vi "DataLog FGV.vi"(7 "Method":T1=enum."Add One Record", 8 "error in (no error)":errorcluster, 10 "length":u16, 11 "New Record":string[](array[string])) -> (0 "error out":errorcluster, 2 "log to file":string[][](array[string]), 3 "Speed Log":string[][](table))   [LabVIEW 2018]
uses:
  Ctls/DatabaseCmd.ctl
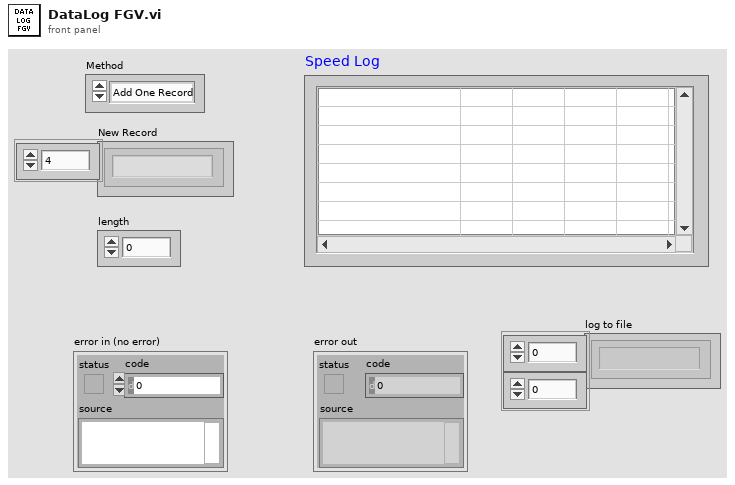
[diagram p1: front panel]
types:
  T1 = typedef "DatabaseCmd.ctl" = enum16{"Insert Table Title", "Add One Record", "Delete Record", "Get Table Records", "Clear"}
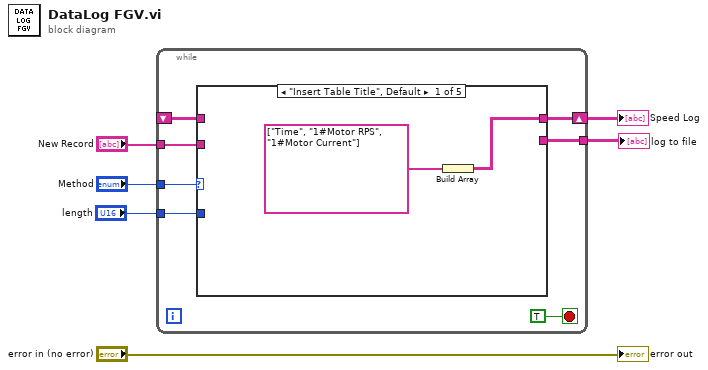
[diagram p0: block diagram]
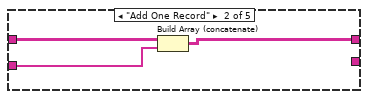
[diagram p2: hidden frame]
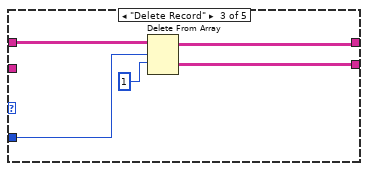
[diagram p3: hidden frame]
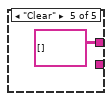
[diagram p5: hidden frame]
diagram:
  n1 = while {
    tunnel: "Method" -> [w12]
    shift-right: [w10] -> w6
    shift-left: _ -> [w11]
    tunnel: "New Record" -> [w9]
    tunnel: "length" -> [w8]
    tunnel: [w7] -> w1
    stop <- TRUE stop-if-true
    n2 = case shown="\"Insert Table Title\", Default" w12 {
      tunnel: w11 -> [_ w16 w23 w24 _]
      tunnel: [w14 w17 w22 w24 string[][] []] -> w10
      tunnel: w9 -> [_ w18 _ _ _]
      tunnel: w8 -> [_ _ w20 _ _]
      tunnel: [_ _ w19 _ _] -> w7
      frame "Insert Table Title", Default {
        n3 = Build Array(string[] ["Time", "1#Motor RPS", "1#Motor Current"]) -> (w14:string[][])
      }
      frame "Add One Record" {
        n4 = Build Array (concatenate)(w16, w18) -> (w17:string[][])
      }
      frame "Delete Record" {
        n5 = Delete From Array(array=w23, length=w20, index (row)=1) -> (deleted portion=w19:string[][], array with subset deleted=w22:string[][])  [unwired: 1 in]
      }
      frame "Get Table Records" {
      }
      frame "Clear" {
      }
    }
  }
  "Speed Log" <- w6
  "log to file" <- w1
  "error out" <- "error in (no error)"
